vi "GetCursorsPositions.vi"(8 "error in (no error)":errorcluster, 10 "Magnification (Microns/Pixel)":T1=1.38 items=["4X"=1.38, "20X"=0.44, "20X_S"=0.32, "50X"=0.034], 11 "Droplets Diameter In":refnum<vi>) -> (0 "error out":errorcluster, 1 "High Limit (microns)":dbl, 2 "Low Limit (microns)":dbl, 3 "Droplets Diameter out":refnum<vi>, 4 "High Limit (Pixels)":dbl, 5 "Low Limit (Pixels)":dbl)   [LabVIEW 2013]
doc: "Use this template to build a VI to use as a subVI."
uses:
  TypeDef/Magnification.ctl
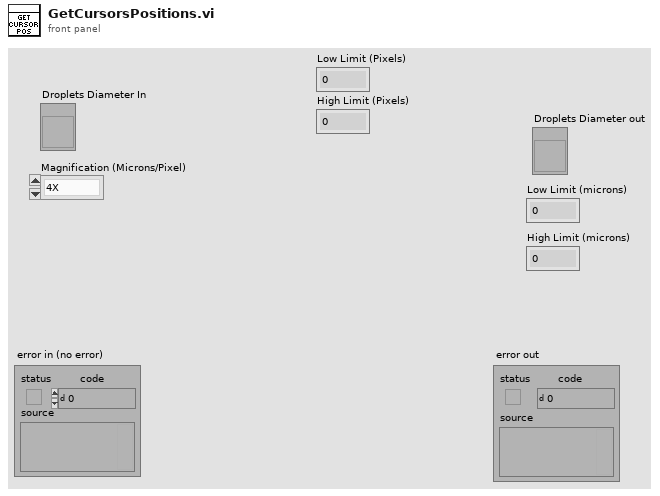
[diagram p1: front panel]
types:
  T1 = typedef "Magnification.ctl" = dbl
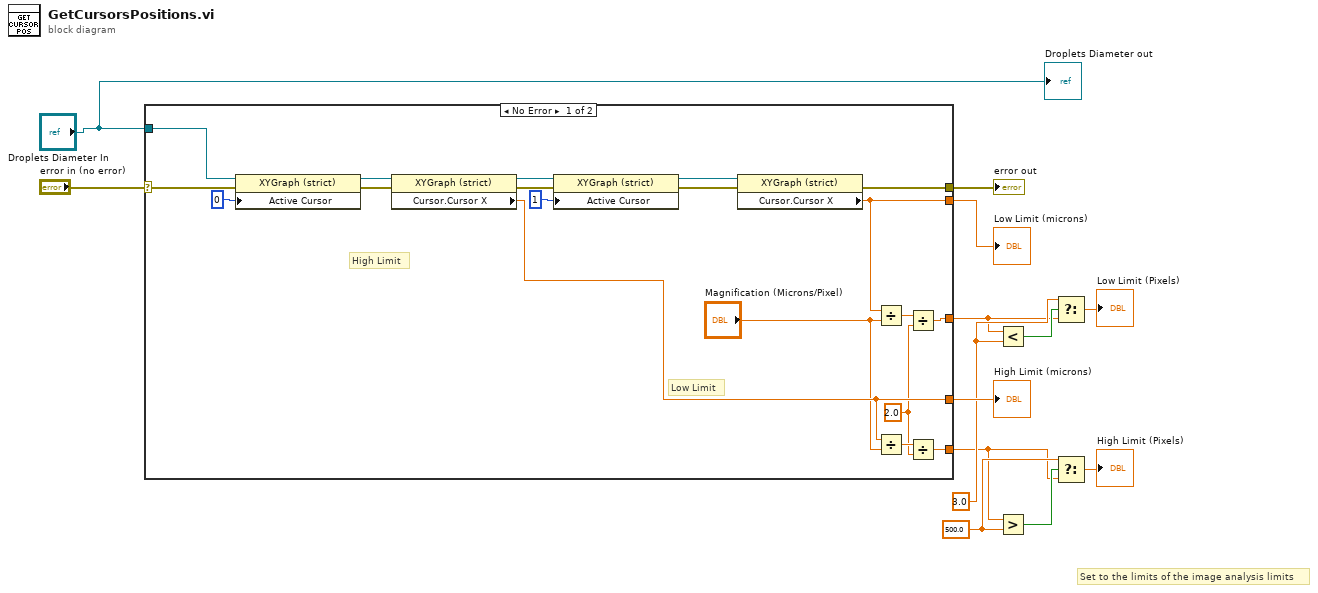
[diagram p0: block diagram]
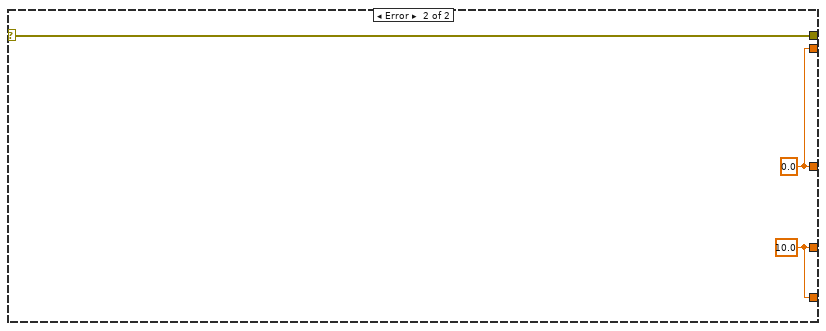
[diagram p2: hidden frame]
diagram:
  w4 = 500.0
  w8 = 3.0
  # "Set to the limits of the image analysis limits"
  n1 = case shown="No Error" "error in (no error)" {
    selector: "error in (no error)" -> [w22 w35]
    tunnel: [w23 w35] -> w12
    tunnel: "Droplets Diameter In" -> [w24 _]
    tunnel: [w21 w33] -> w11
    tunnel: [w19 w34] -> w10
    tunnel: [w17 w33] -> w3
    tunnel: [w14 w34] -> w7
    frame No Error {
      w16 = 2.0
      # "Low Limit"
      # "High Limit"
      n2 = property class="XYGraph (strict)"(reference=w24, error in=w22, "Active Cursor"=u32 0) -> (reference out=w30:refnum<vi>, error out=w28:errorcluster)
      n3 = property class="XYGraph (strict)"(reference=w30, error in=w28) -> (reference out=w29:refnum<vi>, error out=w27:errorcluster, "Cursor.Cursor X"=w21:dbl)
      n4 = property class="XYGraph (strict)"(reference=w29, error in=w27, "Active Cursor"=u32 1) -> (reference out=w26:refnum<vi>, error out=w25:errorcluster)
      n5 = property class="XYGraph (strict)"(reference=w26, error in=w25) -> (error out=w23:errorcluster, "Cursor.Cursor X"=w19:dbl)  [unwired: 1 out]
      n6 = Divide(x=w19, y="Magnification (Microns/Pixel)") -> (x/y=w15:T1)
      n7 = Divide(x=w21, y="Magnification (Microns/Pixel)") -> (x/y=w18:T1)
      n8 = Divide(x=w15, y=w16) -> (x/y=w14:T1)
      n9 = Divide(x=w18, y=w16) -> (x/y=w17:T1)
    }
    frame Error {
      w33 = 10.0 ("Cursor.Cursor X")
      w34 = 0.0 ("Cursor.Cursor X")
    }
  }
  "error out" <- w12
  "Low Limit (microns)" <- w10
  "High Limit (microns)" <- w11
  n10 = Less?(x=w7, y=w8) -> (x < y?=w9:bool)
  n11 = Greater?(x=w3, y=w4) -> (0:w5:bool)
  n12 = Select(t=w8, s=w9, f=w7) -> (s? t:f=→"Low Limit (Pixels)":T1)
  n13 = Select(t=w4, s=w5, f=w3) -> (s? t:f=→"High Limit (Pixels)":T1)
  "Droplets Diameter out" <- "Droplets Diameter In"
